vi "4b_state_sel.vi"(8 "Right":bool, 9 "Left":bool, 10 "Down":bool, 11 "Up":bool) -> (4 "String":string)   [LabVIEW 2012]
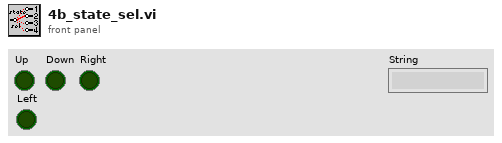
[diagram p1: front panel]
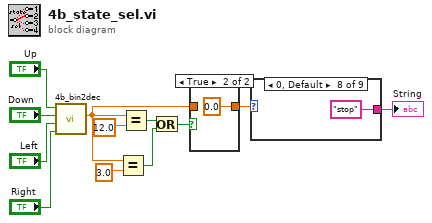
[diagram p0: block diagram]
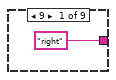
[diagram p2: hidden frame]
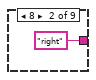
[diagram p3: hidden frame]
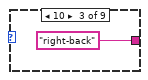
[diagram p4: hidden frame]
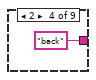
[diagram p5: hidden frame]
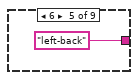
[diagram p6: hidden frame]
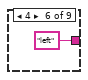
[diagram p7: hidden frame]
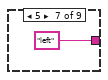
[diagram p8: hidden frame]
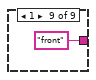
[diagram p9: hidden frame]
diagram:
  n1 = call "4b_bin2dec.vi"("Right"="Right", "Left"="Left", "Down"="Down", "Up"="Up") -> ("Out"=w7:dbl)  [unwired: 7 in]
  n2 = Equal?(x=w7, y=3.0) -> (x = y?=w10:bool)
  n3 = Equal?(x=w7, y=12.0) -> (x = y?=w9:bool)
  n4 = Or(x=w9, y=w10) -> (x .or. y?=w8:bool)
  n5 = case shown="True" w8 {
    tunnel: [w13 0.0 ("Out")] -> w6
    tunnel: w7 -> [w13 _]
    frame False {
    }
    frame True {
    }
  }
  n6 = case shown="0, Default" w6 {
    tunnel: ["right" "right" "right-back" "back" "left-back" "left" "left" "stop" "front"] -> w5
    frame 9 {
    }
    frame 8 {
    }
    frame 10 {
    }
    frame 2 {
    }
    frame 6 {
    }
    frame 4 {
    }
    frame 5 {
    }
    frame 0, Default {
    }
    frame 1 {
    }
  }
  "String" <- w5
